vi "Inject Plug In Value.vi"() -> (5 "Plug in titles":string[](array[string])=["EnFlo Tun:Exit Sound:dB"], 7 "Plug in values":string[](array[string]))   [LabVIEW 2021]
uses:
  Controls/ok_button.ctl
  Controls/Post_Process.ctl
  Controls/Setup.ctl
  Globals/Meas_global.vi
panel:
  in  "OK":T1
  in  "Plug in values 2":string[](array[string])=["41.2"]
  in  "Plug in titles 2":string[](array[string])=["EnFlo Tun:Exit Sound:dB"]
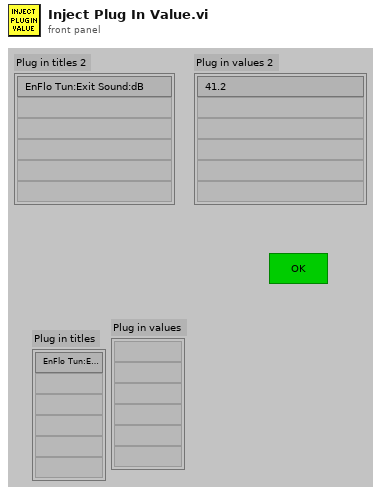
[diagram p1: front panel]
types:
  T1 = typedef "ok_button.ctl" = bool
  T2 = typedef "Setup.ctl" = enum16{"Run Program", "Show Setup", "Save Current Setup", "Setup Front Panel"}
  T3 = typedef "Post_Process.ctl" = enum16{"Take New Data", "Post Process Raw Data File"}
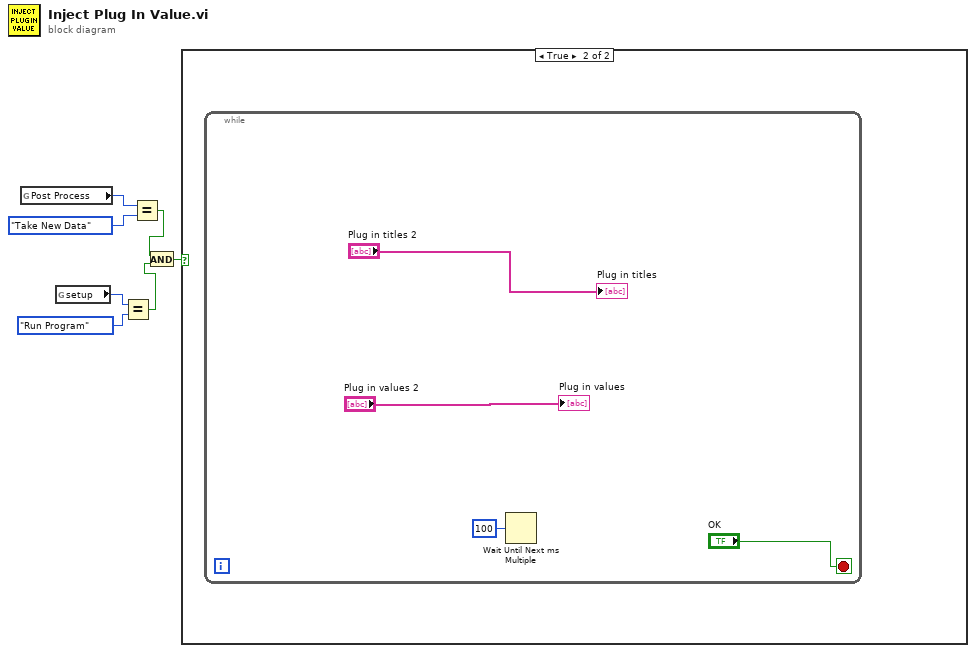
[diagram p0: block diagram]
diagram:
  n1 = global read "Meas_global.vi" "Post Process"() -> (w7:T3)
  n2 = global read "Meas_global.vi" "setup"() -> (w5:T2)
  n3 = Equal?(x=w5, y=Setup."Run Program" ("setup")) -> (x = y?=w2:bool)
  n4 = Equal?(x=w7, y=Post_Process."Take New Data" ("Post Process")) -> (x = y?=w3:bool)
  n5 = And(x=w3, y=w2) -> (x .and. y?=w1:bool)
  n6 = case shown="True" w1 {
    frame False {
    }
    frame True {
      n7 = while {
        stop <- "OK" stop-if-true
        n8 = Wait Until Next ms Multiple(millisecond multiple=u32 100) -> ()  [unwired: 1 out]
        "Plug in values" <- "Plug in values 2"
        "Plug in titles" <- "Plug in titles 2"
      }
    }
  }
